vi "CRYLoad Main Configure.vi"(2 "error in (no error)":errorcluster, 3 "vi reference in":refnum<vi>) -> (0 "error out":errorcluster, 1 "vi reference out":refnum<vi>)   [LabVIEW 2013]
doc: "Config File Reading/Writting\n\nPath \n ini File path\nRWFlag\n 0: no action\n 1: read\n 2: write"
panel:
  out "Array":i32[](array[numeric])
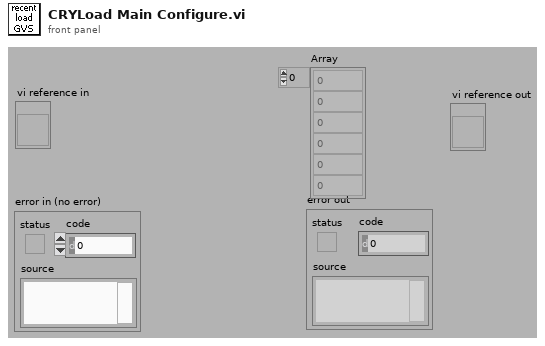
[diagram p1: front panel]
types:
  T1 = cluster{"Section":string, "Items":cluster{"Key":string, "Value":string}[]}[]
  T2 = cluster{"Section":string, "Items":cluster{"Key":string, "Value":string}[]}
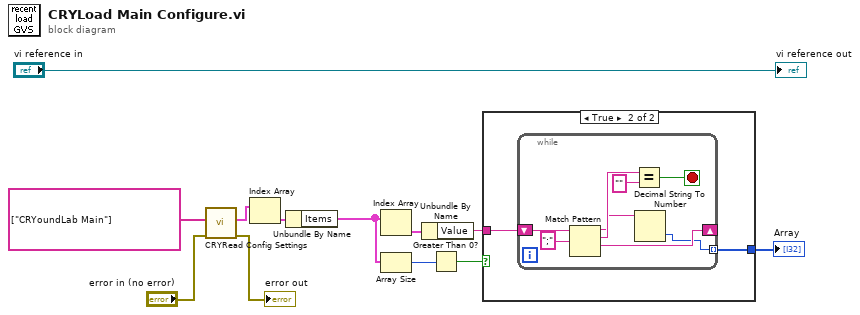
[diagram p0: block diagram]
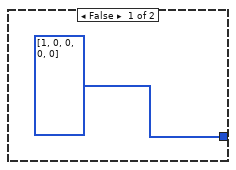
[diagram p2: hidden frame]
diagram:
  n1 = call "CRYRead Config Settings.vi"("error in (no error)"="error in (no error)", "Section"=string[] ["CRYoundLab Main"]) -> ("error out"=→"error out":errorcluster, "Configuration Data"=w2:T1)  [unwired: 8 out]
  n2 = Index Array(array=w2) -> (element=w1:T2)  [unwired: 1 in]
  n3 = Unbundle By Name(w1) -> ("Items"=w11:cluster{"Key":string, "Value":string}[])
  n4 = Index Array(array=w11) -> (element=w8:cluster{"Key":string, "Value":string})  [unwired: 1 in]
  n5 = Array Size(array=w11) -> (size(s)=w10:i32)
  n6 = Unbundle By Name(w8) -> ("Value"=w7:string)
  n7 = Greater Than 0?(x=w10) -> (x > 0?=w9:bool)
  n8 = case shown="True" w9 {
    tunnel: w7 -> [_ w15]
    tunnel: [i32[] [1, 0, 0, 0, 0] w14] -> w5
    frame False {
    }
    frame True {
      n9 = while {
        shift-right: [w22] -> _
        shift-left: w15 -> [w20]
        tunnel: [w17] -> w14 mode=indexing
        stop <- w18 stop-if-true
        n10 = Match Pattern(string=w20, regular expression=";" ("search string")) -> (before substring=w16:string, match substring=w19:string, after substring=w22:string)  [unwired: 2 out]
        n11 = Equal?(x=w19, y="") -> (x = y?=w18:bool)
        n12 = Decimal String To Number(string=w16) -> (number=w17:i32)  [unwired: 3 out]
      }
    }
  }
  "Array" <- w5
  "vi reference out" <- "vi reference in"
